vi "外观 2.vi"(0 "Data In":T9 caption="数据输入" {"数值" format="%04x"}, 2 "Display State In":T7 caption="显示状态输入" {"值" items=["三通阀", "排阀"]}, 3 "Container State":T8 caption="容器状态") -> (6 "Data Out":T9 caption="数据输出" {"数值" format="%04x"}, 7 "Display State Out":T7 caption="显示状态输出" {"值" items=["三通阀", "排阀"]}, 8 "Action":T6 caption="动作")   [LabVIEW 2016, in "CODMn调试控件V3.xctl"]
uses:
  <vilib>/_xctls/Container State.ctl
  <vilib>/_xctls/Action.ctl
  <vilib>/_xctls/XControlSupport.lvlib
panel:
  in  "反应杯温度控制:":u16
  in  "偏心轮抽取液体次数:":u16
  in  "缺液检测":bool caption="V2"
  in  "偏心轮:":u16 caption="mL"
  in  "模式":enum32{"测试模式", "流程模式"}(tab)
  in  "外设:":T1
  in  "加热:":bool caption="V2"
  in  "摄氏度":u16
  in  "量:":u16=5000
  in  "注射泵:":T2(radio)
  in  "进样:":T3(radio)
  out "阀配置":u8(ring) items=["三通阀", "排阀"]
  in  "柱塞泵体积/等待时间":u16=5000
  in  "功能选择":enum32{"等待", "复位", "注入", "注出"}(radio)=enum."注入"
  out "字符串":string="柱塞泵体积μL"
  in  "外设":T4
  in  "其他":enum32{"未选择", "更新A值", "更新B值", "反滴定"}(radio)
  in  "阀口选择":T5(radio)
  # "次(0代表不动作)"
  # "℃(0代表不控温)"
  # "uL"
  # "℃"
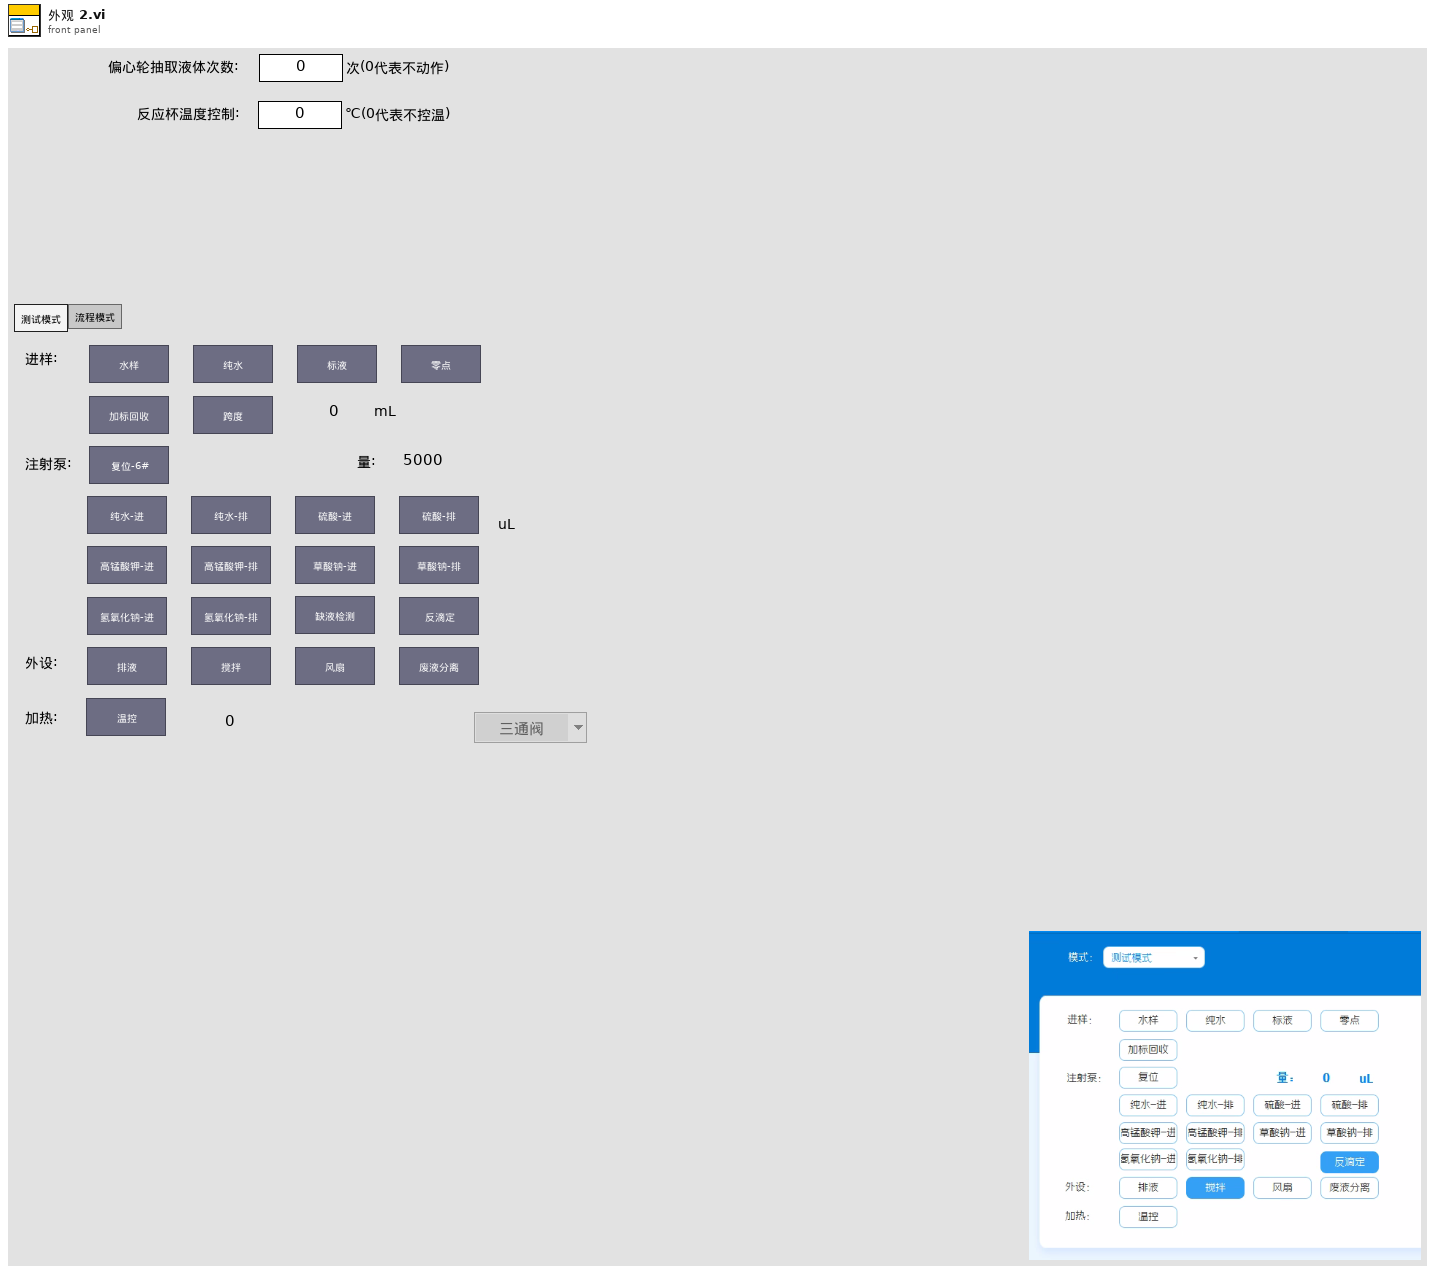
[diagram p1: front panel]
types:
  T1 = cluster{"排液":bool, "搅拌":bool, "风扇":bool, "废液分离":bool}
  T2 = enum32{"未选择", "纯水-进", "纯水-排", "硫酸-进", "硫酸-排", "复位", "高锰酸钾-进", "高锰酸钾-排", "草酸钠-进", "草酸钠-排", "氢氧化钠-进", "氢氧化钠-排", "反滴定"}
  T3 = enum32{"未选择", "水样", "纯水", "标液", "零点", "加标回收", "跨度"}
  T4 = cluster{"排液阀":bool, "搅拌":bool, "冷凝风扇":bool, "废液分离阀":bool, "电磁阀1":bool, "电磁阀2":bool, "电磁阀3":bool, "电磁阀4":bool, "电磁阀5":bool, "电磁阀6":bool, "电磁阀7":bool}
  T5 = enum32{"未选择", "V1", "V2", "V3", "V4", "V5", "V6", "V7", "V8", "V9", "V10", "V11", "V12"}
  T6 = typedef "XControlSupport.lvlib/Action.ctl" = cluster{"Data Changed?":bool, "State Changed?":bool, "Action Name":string}
  T7 = typedef "CODMn调试控件V3.xctl/状态 2.ctl" = cluster{"值":u8}
  T8 = typedef "XControlSupport.lvlib/Container State.ctl" = cluster{"Indicator?":bool, "Run Mode?":bool, " Refnum":refnum<vi>}
  T9 = typedef "CODMn调试控件V3.xctl/数据 2.ctl" = cluster{"数值":u16[], "模式":enum32{"测试模式", "流程模式"}}
  T10 = enum32{"未选择", "水样", "纯水", "标液", "零点", "加标回收", "加标回收 2"}
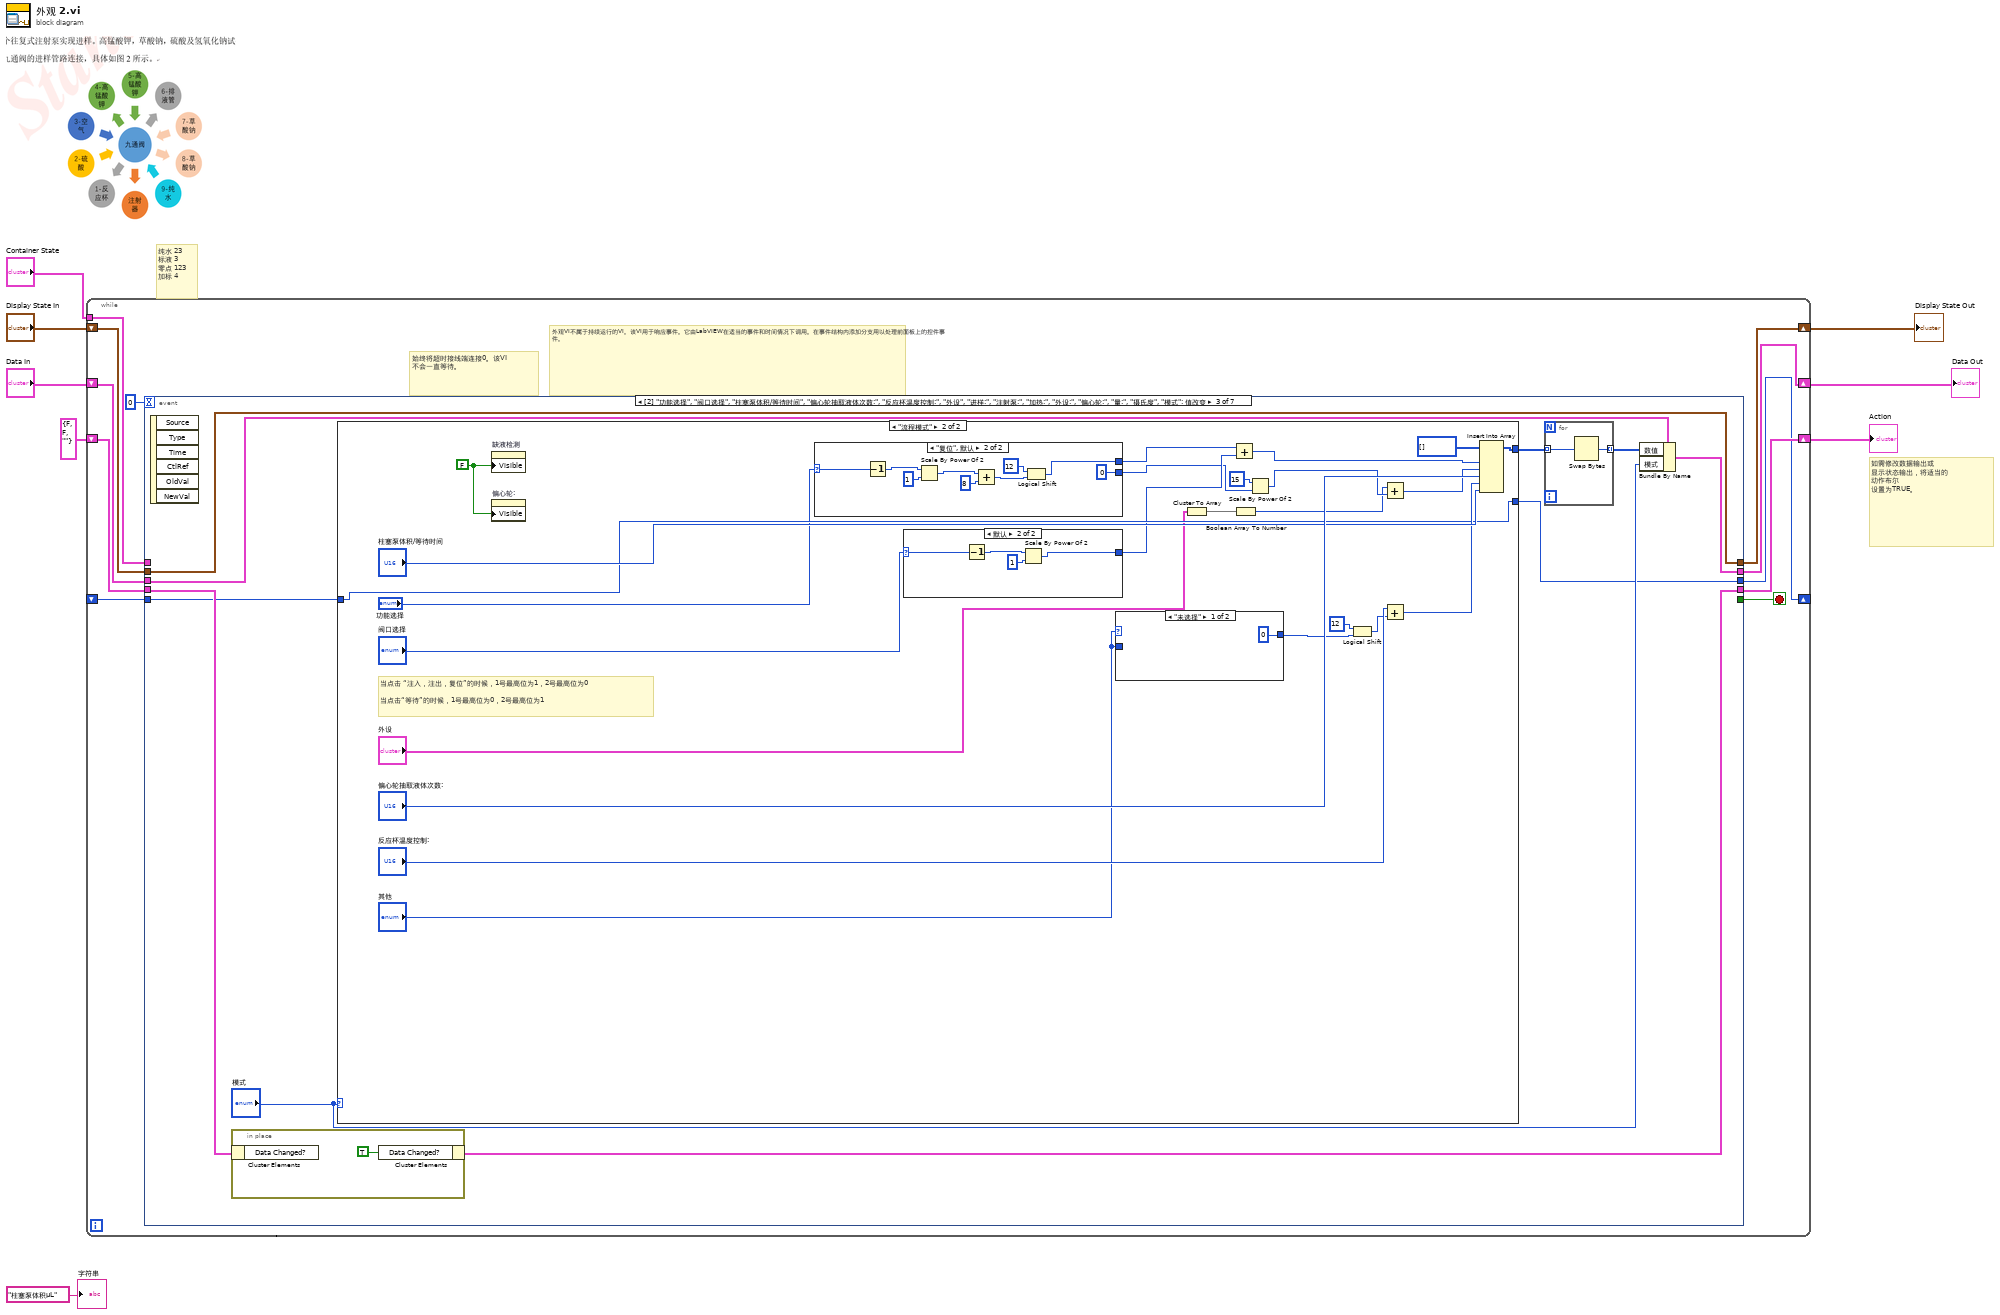
[diagram p0: block diagram]
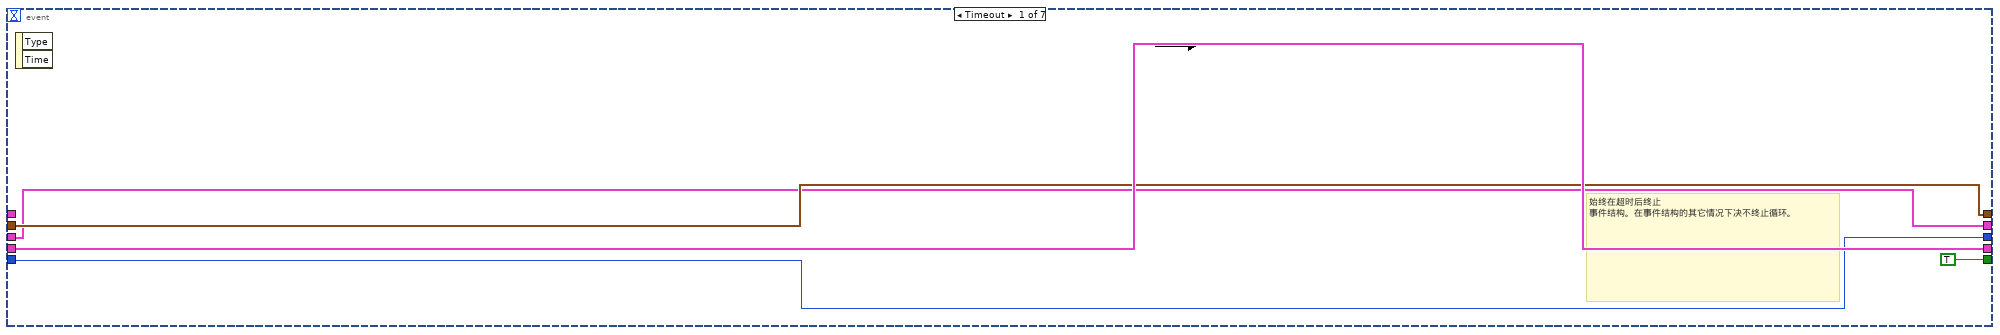
[diagram p2: hidden frame]
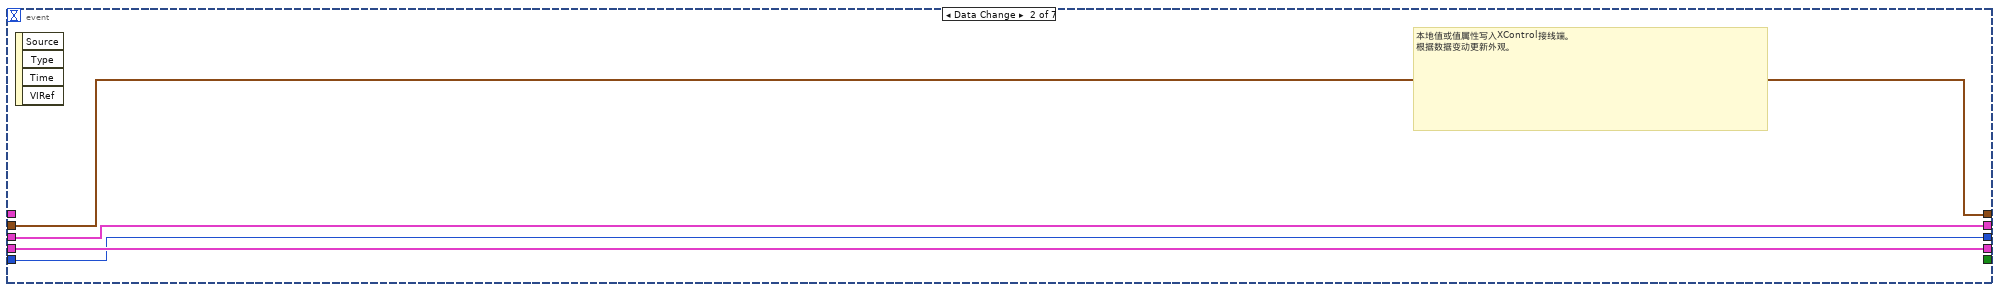
[diagram p3: hidden frame]
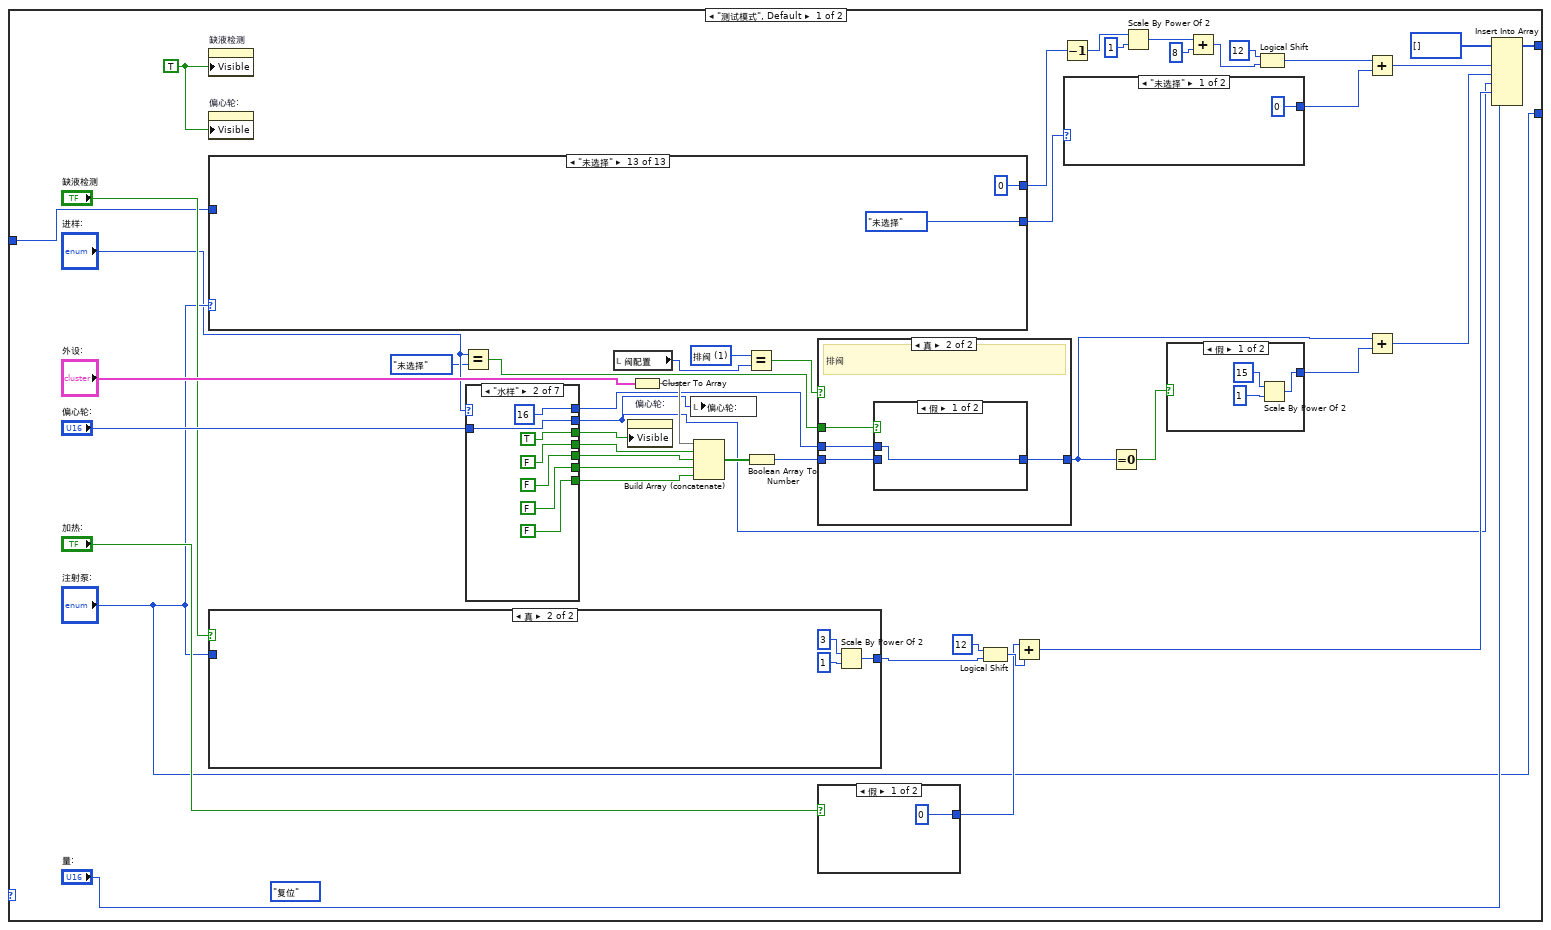
[diagram p4: hidden frame]
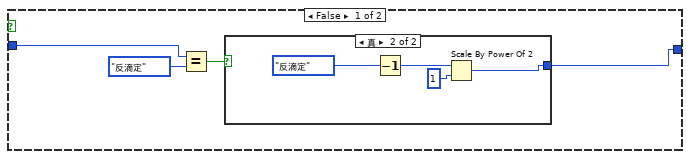
[diagram p7: hidden frame]
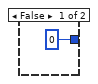
[diagram p8: hidden frame]
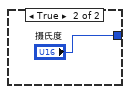
[diagram p9: hidden frame]
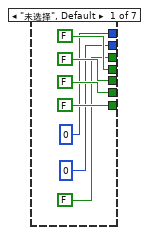
[diagram p10: hidden frame]
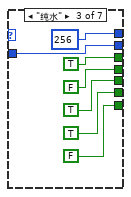
[diagram p11: hidden frame]
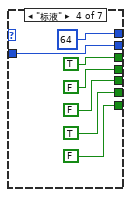
[diagram p12: hidden frame]
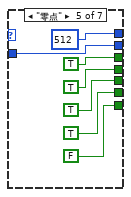
[diagram p13: hidden frame]
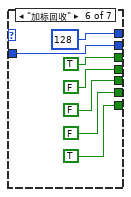
[diagram p14: hidden frame]
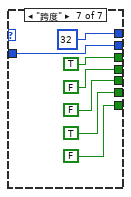
[diagram p15: hidden frame]
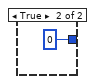
[diagram p16: hidden frame]
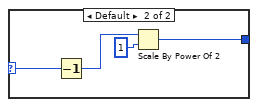
[diagram p17: hidden frame]
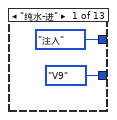
[diagram p18: hidden frame]
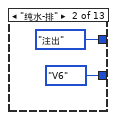
[diagram p19: hidden frame]
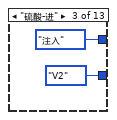
[diagram p20: hidden frame]
diagram:
  # "纯水 23\n标液 3\n零点 123\n加标 4"
  # "如需修改数据输出或\n显示状态输出，将适当的\n动作布尔\n设置为TRUE。"
  n1 = while {
    shift-right: [w18] -> w5
    shift-left: "Display State In" -> [w19]
    tunnel: "Container State" -> [w15]
    shift-right: [w13] -> w8
    shift-left: "Data In" -> [w14]
    shift-right: [w11] -> w3
    shift-left: T6 {"Data Changed?"=FALSE, "State Changed?"=FALSE, "Action Name"=""} ("Action") -> [w12]
    shift-right: [w10] -> _
    shift-left: _ -> [w9]
    stop <- w17 stop-if-true
    # "外观VI不属于持续运行的VI。该VI用于响应事件。它由LabVIEW在适当的事件和时间情况下调用。在事件结构内添加分支用以处理前面板上的控件事件。"
    # "始终将超时接线端连接0。该VI\n不会一直等待。"
    n2 = event shown="[2] \"功能选择\", \"阀口选择\", \"柱塞泵体积/等待时间\", \"偏心轮抽取液体次数:\", \"反应杯温度控制:\", \"外设\", \"进样:\", \"注射泵:\", \"加热:\", \"外设:\", \"偏心轮:\", \"量:\", \"摄氏度\", \"模式\": 值改变" {
      selector: _ -> [_ _ _ _ _ _ _]
      dyn-events: _ -> [_ _ _ _ _ _ _]
      timeout: 0 -> [_ _ _ _ _ _ _]
      tunnel: w19 -> [w22 w25 w38 w299 w300 w308 w312]
      tunnel: [w22 w25 w38 w299 w300 w308 w312] -> w18
      tunnel: [TRUE _ _ _ _ _ _] -> w17
      tunnel: w15 -> [_ _ _ _ _ w309 w314]
      tunnel: w14 -> [w21 w28 w34 w298 w304 w307 w311]
      tunnel: [w21 w28 w31 w298 w304 w307 w311] -> w13
      tunnel: [w23 w27 w36 w297 w303 w306 w310] -> w11
      tunnel: w12 -> [w23 w27 w37 w297 w303 w306 w310]
      tunnel: [w20 w26 w30 w292 w302 w305 w313] -> w10
      tunnel: w9 -> [w20 w26 w29 w292 w302 w305 w313]
      event Timeout {
        # "始终在超时后终止\n事件结构。在事件结构的其它情况下决不终止循环。"
        n3 = event-data() -> ()  [unwired: 1 in, 2 out]
      }
      event Data Change {
        # "本地值或值属性写入XControl接线端。\n根据数据变动更新外观。"
        n4 = event-data() -> ()  [unwired: 1 in, 4 out]
      }
      event "功能选择", "阀口选择", "柱塞泵体积/等待时间", "偏心轮抽取液体次数:", "反应杯温度控制:", "外设", "进样:", "注射泵:", "加热:", "外设:", "偏心轮:", "量:", "摄氏度", "模式": Value Change {
        n5 = event-data() -> ()  [unwired: 1 in, 6 out]
        n6 = in-place {
          n7 = in-place-cluster #1(w37) -> ()  [unwired: 1 out]
          n8 = in-place-cluster #1("Data Changed?"=TRUE) -> (w36:T6)
        }
        n9 = case shown="\"流程模式\"" "模式" {
          tunnel: [w62 w262] -> w35
          tunnel: ["注射泵:" w256] -> w30
          tunnel: w29 -> [w49 w256]
          frame "测试模式", Default {
            w39 = TRUE ("可见")
            w43 = u8 1 items=["三通阀", "排阀"] ("Value")
            (unwired) enum32{"等待", "复位", "注入", "注出"}."复位" ("功能选择")
            n10 = property on="缺液检测" class="Bool (严格)"("Visible"=w39) -> ()  [unwired: 2 in, 2 out]
            n11 = property on="偏心轮:" class="DigNum (严格)"("Visible"=w39) -> ()  [unwired: 2 in, 2 out]
            n12 = case shown="\"未选择\"" "注射泵:" {
              tunnel: [enum32{"等待", "复位", "注入", "注出"}."注入" ("功能选择") enum32{"等待", "复位", "注入", "注出"}."注出" ("功能选择") enum32{"等待", "复位", "注入", "注出"}."注入" ("功能选择") enum32{"等待", "复位", "注入", "注出"}."注出" ("功能选择") enum32{"等待", "复位", "注入", "注出"}."复位" ("功能选择") enum32{"等待", "复位", "注入", "注出"}."注入" ("功能选择") enum32{"等待", "复位", "注入", "注出"}."注出" ("功能选择") enum32{"等待", "复位", "注入", "注出"}."注入" ("功能选择") enum32{"等待", "复位", "注入", "注出"}."注出" ("功能选择") enum32{"等待", "复位", "注入", "注出"}."注入" ("功能选择") enum32{"等待", "复位", "注入", "注出"}."注出" ("功能选择") 0 0] -> w61
              tunnel: [T5."V9" ("阀口选择") T5."V6" ("阀口选择") T5."V2" ("阀口选择") T5."V1" ("阀口选择") T5."V6" ("阀口选择") T5."V5" ("阀口选择") T5."V4" ("阀口选择") T5."V7" ("阀口选择") T5."V8" ("阀口选择") T5."V3" ("阀口选择") T5."V6" ("阀口选择") T5."未选择" ("阀口选择") T5."未选择" ("阀口选择")] -> w82
              tunnel: w49 -> [_ _ _ _ _ w174 w183 w192 w207 w222 w231 _ _]
              frame "纯水-进" {
              }
              frame "纯水-排" {
              }
              frame "硫酸-进" {
              }
              frame "硫酸-排" {
              }
              frame "复位" {
              }
              frame "高锰酸钾-进" {
                n13 = Greater Or Equal?(x=w174, y=T2."草酸钠-进" ("注射泵:")) -> (x >= y?=w177:bool)
                n14 = Less Or Equal?(x=w174, y=T2."氢氧化钠-排" ("注射泵:")) -> (x <= y?=w178:bool)
                n15 = And(x=w177, y=w178) -> (x .and. y?=w179:bool)
                n16 = case shown="真" w179 {
                  frame False {
                  }
                  frame True {
                    n17 = One Button Dialog(message="“\"警告:未进行润洗\n或者进出液不匹配\"”" ("消息")) -> ()  [unwired: 1 in, 1 out]
                  }
                }
              }
              frame "高锰酸钾-排" {
                n18 = Greater Or Equal?(x=w183, y=T2."草酸钠-进" ("注射泵:")) -> (x >= y?=w186:bool)
                n19 = Less Or Equal?(x=w183, y=T2."氢氧化钠-排" ("注射泵:")) -> (x <= y?=w187:bool)
                n20 = And(x=w186, y=w187) -> (x .and. y?=w188:bool)
                n21 = case shown="真" w188 {
                  frame False {
                  }
                  frame True {
                    n22 = One Button Dialog(message="“\"警告:未进行润洗\n或者进出液不匹配\"”" ("消息")) -> ()  [unwired: 1 in, 1 out]
                  }
                }
              }
              frame "草酸钠-进" {
                n23 = Greater Or Equal?(x=w192, y=T2."氢氧化钠-进" ("注射泵:")) -> (x >= y?=w195:bool)
                n24 = Less Or Equal?(x=w192, y=T2."氢氧化钠-排" ("注射泵:")) -> (x <= y?=w194:bool)
                n25 = Greater Or Equal?(x=w192, y=T2."高锰酸钾-进" ("注射泵:")) -> (x >= y?=w200:bool)
                n26 = Less Or Equal?(x=w192, y=T2."高锰酸钾-排" ("注射泵:")) -> (x <= y?=w201:bool)
                n27 = And(x=w195, y=w194) -> (x .and. y?=w193:bool)
                n28 = And(x=w200, y=w201) -> (x .and. y?=w202:bool)
                n29 = Or(x=w193, y=w202) -> (x .or. y?=w203:bool)
                n30 = case shown="真" w203 {
                  frame False {
                  }
                  frame True {
                    n31 = One Button Dialog(message="“\"警告:未进行润洗\n或者进出液不匹配\"”" ("消息")) -> ()  [unwired: 1 in, 1 out]
                  }
                }
              }
              frame "草酸钠-排" {
                n32 = Greater Or Equal?(x=w207, y=T2."氢氧化钠-进" ("注射泵:")) -> (x >= y?=w210:bool)
                n33 = Less Or Equal?(x=w207, y=T2."氢氧化钠-排" ("注射泵:")) -> (x <= y?=w209:bool)
                n34 = Greater Or Equal?(x=w207, y=T2."高锰酸钾-进" ("注射泵:")) -> (x >= y?=w215:bool)
                n35 = Less Or Equal?(x=w207, y=T2."高锰酸钾-排" ("注射泵:")) -> (x <= y?=w216:bool)
                n36 = And(x=w210, y=w209) -> (x .and. y?=w208:bool)
                n37 = And(x=w215, y=w216) -> (x .and. y?=w217:bool)
                n38 = Or(x=w208, y=w217) -> (x .or. y?=w218:bool)
                n39 = case shown="真" w218 {
                  frame False {
                  }
                  frame True {
                    n40 = One Button Dialog(message="“\"警告:未进行润洗\n或者进出液不匹配\"”" ("消息")) -> ()  [unwired: 1 in, 1 out]
                  }
                }
              }
              frame "氢氧化钠-进" {
                n41 = Less Or Equal?(x=w222, y=T2."草酸钠-排" ("注射泵:")) -> (x <= y?=w227:bool)
                n42 = Greater Or Equal?(x=w222, y=T2."高锰酸钾-进" ("注射泵:")) -> (x >= y?=w226:bool)
                n43 = And(x=w226, y=w227) -> (x .and. y?=w223:bool)
                n44 = case shown="真" w223 {
                  frame False {
                  }
                  frame True {
                    n45 = One Button Dialog(message="“\"警告:未进行润洗\n或者进出液不匹配\"”" ("消息")) -> ()  [unwired: 1 in, 1 out]
                  }
                }
              }
              frame "氢氧化钠-排" {
                n46 = Less Or Equal?(x=w231, y=T2."草酸钠-排" ("注射泵:")) -> (x <= y?=w236:bool)
                n47 = Greater Or Equal?(x=w231, y=T2."高锰酸钾-进" ("注射泵:")) -> (x >= y?=w235:bool)
                n48 = And(x=w235, y=w236) -> (x .and. y?=w232:bool)
                n49 = case shown="真" w232 {
                  frame False {
                  }
                  frame True {
                    n50 = One Button Dialog(message="“\"警告:未进行润洗\n或者进出液不匹配\"”" ("消息")) -> ()  [unwired: 1 in, 1 out]
                  }
                }
              }
              frame "反滴定" {
              }
              frame "未选择" {
              }
            }
            n51 = case shown="真" "缺液检测" {
              tunnel: "注射泵:" -> [w94 _]
              tunnel: [w92 w102] -> w64
              frame False {
                n52 = Equal?(x=w94, y=T2."反滴定" ("注射泵:")) -> (x = y?=w93:bool)
                n53 = case shown="真" w93 {
                  tunnel: [i16 0 w97] -> w92
                  frame False {
                  }
                  frame True {
                    n54 = Decrement(x=enum32{"未选择", "更新A值", "更新B值", "反滴定"}."反滴定" ("其他")) -> (x-1=w98:enum32{"未选择", "更新A值", "更新B值", "反滴定"})
                    n55 = Scale By Power Of 2(n=w98, x=i16 1 ("y")) -> (x*2^n=w97:i16)
                  }
                }
              }
              frame True {
                n56 = Scale By Power Of 2(n=i16 3, x=i16 1 ("y")) -> (x*2^n=w102:i16)
              }
            }
            n57 = Equal?(x="进样:", y=T10."未选择") -> (x = y?=w41:bool)
            n58 = case shown="\"水样\"" "进样:" {
              tunnel: [FALSE FALSE FALSE FALSE TRUE FALSE FALSE] -> w76
              tunnel: [FALSE FALSE TRUE FALSE TRUE FALSE FALSE] -> w75
              tunnel: [FALSE FALSE TRUE TRUE TRUE FALSE TRUE] -> w74
              tunnel: [FALSE FALSE FALSE FALSE FALSE TRUE FALSE] -> w73
              tunnel: "偏心轮:" -> [_ w115 w122 w129 w136 w143 w153]
              tunnel: [u16 0 ("偏心轮:") w115 w122 w129 w136 w143 w153] -> w59
              tunnel: [FALSE TRUE TRUE TRUE TRUE TRUE TRUE] -> w58
              tunnel: [u16 0 ("数字") u16 16 ("数字") u16 256 ("数字") u16 64 ("数字") u16 512 ("数字") u16 128 ("数字") u16 32 ("数字")] -> w44
              frame "未选择", Default {
              }
              frame "水样" {
              }
              frame "纯水" {
              }
              frame "标液" {
              }
              frame "零点" {
              }
              frame "加标回收" {
              }
              frame "跨度" {
              }
            }
            n59 = local read "阀配置"() -> (w42:u8)
            n60 = property on="偏心轮:" class="DigNum (严格)"("Visible"=w58) -> ()  [unwired: 2 in, 2 out]
            n61 = Cluster To Array(cluster="外设:") -> (array=w77:bool[])
            n62 = local write "偏心轮:"(w59) -> ()
            n63 = Build Array (concatenate)(w77, w76, w75, w74, w73) -> (w72:bool[])
            n64 = Equal?(x=w43, y=w42) -> (x = y?=w40:bool)
            n65 = Boolean Array To Number ("布尔数组至数值转换")(Boolean array=w72) -> (number=w46:u16)
            n66 = case shown="真" w40 {
              tunnel: w46 -> [w85 w89]
              tunnel: [w85 w88] -> w45
              tunnel: w44 -> [_ w87]
              tunnel: w41 -> [_ w86]
              frame False {
              }
              frame True {
                # "排阀"
                n67 = case shown="假" w86 {
                  tunnel: w89 -> [_ w91]
                  tunnel: [w90 w91] -> w88
                  tunnel: w87 -> [w90 _]
                  frame False {
                  }
                  frame True {
                  }
                }
              }
            }
            n68 = case shown="假" "加热:" {
              tunnel: [u16 0 ("摄氏度") "摄氏度"] -> w65
              frame False {
              }
              frame True {
              }
            }
            n69 = Logical Shift(y=i16 12, x=w64) -> (x << y=w66:i16)
            n70 = Add(x=w65, y=w66) -> (x+y=w63:u16)
            n71 = Decrement(x=w61) -> (x-1=w52:u32)
            n72 = case shown="\"未选择\"" w82 {
              selector: w82 -> [_ w161]
              tunnel: [i16 0 ("y") w163] -> w84
              frame "未选择" {
              }
              frame Default {
                n73 = Decrement(x=w161) -> (x-1=w162:T5)
                n74 = Scale By Power Of 2(n=w162, x=i16 1 ("y")) -> (x*2^n=w163:i16)
              }
            }
            n75 = Equal To 0?(x=w45) -> (x = 0?=w79:bool)
            n76 = Scale By Power Of 2(n=w52, x=i16 1 ("y")) -> (x*2^n=w55:i16)
            n77 = case shown="假" w79 {
              tunnel: [w155 u16 0] -> w80
              frame False {
                n78 = Scale By Power Of 2(n=i16 15, x=u16 1 ("y")) -> (x*2^n=w155:u16)
              }
              frame True {
              }
            }
            n79 = Add(x=w55, y=i16 8) -> (x+y=w56:i16)
            n80 = Logical Shift(y=i16 12, x=w56) -> (x << y=w83:i16)
            n81 = Add(x=w83, y=w84) -> (x+y=w71:i16)
            n82 = Add(x=w45, y=w80) -> (x+y=w70:u16)
            n83 = Insert Into Array(array=u16[] [] ("数组"), new element #1=w71, new element #2=w70, new element #3=w59, new element #4=w63, new element #5="量:") -> (w62:u16[])  [unwired: 1 in]
          }
          frame "流程模式" {
            w255 = FALSE ("可见")
            # "当点击 “注入，注出，复位”的时候，1号最高位为1，2号最高位为0\n\n当点击“等待”的时候，1号最高位为0，2号最高位为1"
            n84 = property on="缺液检测" class="Bool (严格)"("Visible"=w255) -> ()  [unwired: 2 in, 2 out]
            n85 = property on="偏心轮:" class="DigNum (严格)"("Visible"=w255) -> ()  [unwired: 2 in, 2 out]
            n86 = case shown="\"复位\", 默认" "功能选择" {
              selector: "功能选择" -> [_ w271]
              tunnel: [u16 1 ("y") u16 0 ("y")] -> w246
              tunnel: [i16 0 ("y") w270] -> w245
              frame "等待" {
              }
              frame "复位", Default {
                n87 = Decrement(x=w271) -> (x-1=w272:enum32{"等待", "复位", "注入", "注出"})
                n88 = Scale By Power Of 2(n=w272, x=i16 1 ("y")) -> (x*2^n=w275:i16)
                n89 = Add(x=w275, y=i16 8) -> (x+y=w274:i16)
                n90 = Logical Shift(y=i16 12, x=w274) -> (x << y=w270:i16)
              }
            }
            n91 = case shown="默认" "阀口选择" {
              selector: "阀口选择" -> [_ w281]
              tunnel: [i16 0 ("y") w283] -> w254
              frame "未选择" {
              }
              frame Default {
                n92 = Decrement(x=w281) -> (x-1=w282:T5)
                n93 = Scale By Power Of 2(n=w282, x=i16 1 ("y")) -> (x*2^n=w283:i16)
              }
            }
            n94 = case shown="\"未选择\"" "其他" {
              tunnel: "其他" -> [_ w286]
              tunnel: [i16 0 w285] -> w259
              frame "未选择" {
              }
              frame "更新A值", Default {
                n95 = Decrement(x=w286) -> (x-1=w288:enum32{"未选择", "更新A值", "更新B值", "反滴定"})
                n96 = Scale By Power Of 2(n=w288, x=i16 1 ("y")) -> (x*2^n=w285:i16)
              }
            }
            n97 = Cluster To Array(cluster="外设") -> (array=w248:bool[])
            n98 = Add(x=w245, y=w254) -> (x+y=w252:i16)
            n99 = Boolean Array To Number ("布尔数组至数值转换")(Boolean array=w248) -> (number=w250:u16)
            n100 = Scale By Power Of 2(n=i16 15, x=w246) -> (x*2^n=w251:u16)
            n101 = Logical Shift(y=i16 12, x=w259) -> (x << y=w258:i16)
            n102 = Add(x=w250, y=w251) -> (x+y=w261:u16)
            n103 = Add(x="反应杯温度控制:", y=w258) -> (x+y=w263:u16)
            n104 = Insert Into Array(array=u16[] [] ("数组"), new element #1=w252, new element #2=w261, new element #3="偏心轮抽取液体次数:", new element #4=w263, new element #5="柱塞泵体积/等待时间") -> (w262:u16[])  [unwired: 1 in]
          }
        }
        n105 = for {
          tunnel: w35 -> [w290] mode=indexing
          tunnel: [w289] -> w33 mode=indexing
          n106 = Swap Bytes(anything=w290) -> (byte swapped=w289:u16)
        }
        n107 = Bundle By Name(cluster=w34, "数值"=w33, "模式"="模式") -> (w31:T9)
      }
      event "柱塞泵体积/等待时间", "偏心轮抽取液体次数:", "反应杯温度控制:", "偏心轮:", "量:", "摄氏度": Mouse Down {
        n108 = event-data() -> ("CtlRef"=w296:refnum<vi>)  [unwired: 1 in, 7 out]
        n109 = property class="DigNum (严格)"(reference=w296) -> (reference out=w295:refnum<vi>, "Value"=w294:u16)  [unwired: 1 in, 1 out]
        n110 = call "数字键盘.vi"("OldNumber"=w294) -> ("NewNumber"=w293:sgl)
        n111 = property class="DigNum (严格)"(reference=w295, "Val(Sgnl)"=w293) -> ()  [unwired: 1 in, 2 out]
      }
      event Display State Change {
        # "拖放该XControl的新实例、复制、撤消操作或者在XControl内执行自定义属性或方法均可改变显示状态。更新相应外观。"
        n112 = event-data() -> ()  [unwired: 1 in, 4 out]
        n113 = Unbundle By Name(w300) -> ("值"=→"阀配置":u8)
      }
      event Direction Change {
        # "XControl的方向由输入控件转换为显示控件，反之亦然。更新相应外观。"
        n114 = event-data() -> ()  [unwired: 1 in, 4 out]
        n115 = Unbundle By Name(w309) -> ()  [unwired: 1 out]
      }
      event Exec State Change {
        # "包含该XControl的VI已从编辑模式切换至运行模式，反之亦然。\n相应的更新外观。"
        # "分别处理编辑模式和\n运行模式"
        n116 = event-data() -> ()  [unwired: 1 in, 4 out]
        n117 = Unbundle By Name(w314) -> ()  [unwired: 1 out]
      }
    }
  }
  "Display State Out" <- w5
  "Data Out" <- w8
  "Action" <- w3
  "字符串" <- "柱塞泵体积μL" ("字符串")
